vi "Configure Burst.vi"(7 "Channel (1:Chan A)":i32(ring)=1 items=["System (To)", "Channel A", "Channel B", "Channel C", "Channel D", "Channel E", "Channel F", "Channel G", "Channel H"], 8 "error in (no error)":errorcluster, 10 "Burst # (10)":i32=10, 11 "VISA resource name":refnum<visa-resource-name>) -> (0 "error out":errorcluster, 3 "VISA resource name out":refnum<visa-resource-name>)   [LabVIEW 2019, in "Quantum Composers 9000 Series.lvlib"]
doc: "This VI is used to configure the burst mode of operation for a channel or the system timer (To)."
uses:
  Quantum Composers 9000 Series.lvlib
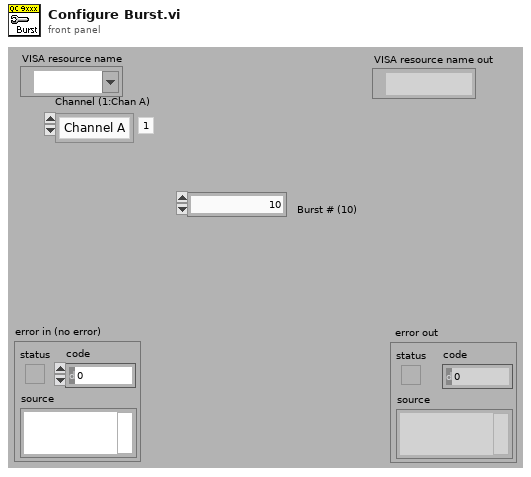
[diagram p1: front panel]
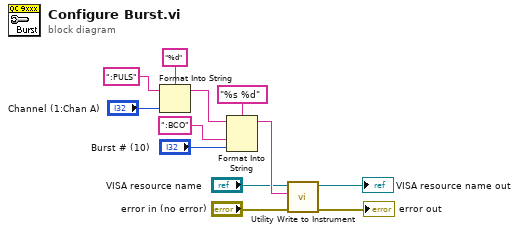
[diagram p0: block diagram]
diagram:
  n1 = Format Into String(format string="%d", initial string=":PULS", "Channel (1:Chan A)") -> (resulting string=w1:string)  [unwired: 1 in, 1 out]
  n2 = Format Into String(format string="%s %d", initial string=w1, ":BCO", "Burst # (10)") -> (resulting string=w6:string)  [unwired: 1 in, 1 out]
  n3 = call "Utility Write to Instrument.vi"("error in (no error)"="error in (no error)", "Write Buffer"=w6, "VISA resource name"="VISA resource name") -> ("error out"=→"error out":errorcluster, "VISA resource name out"=→"VISA resource name out":refnum<visa-resource-name>)  [unwired: 6 in, 1 out]
